vi "DeleteDVR.vi"(8 "error in (no error)":errorcluster, 10 "Error Return Notifier":refnum<notifier>, 11 "IAmGLF To Create DVR":refnum<class "IAmGLF.lvclass">) -> (0 "error out":errorcluster)   [LabVIEW 2024, in "GLF.lvlib" / "DVRHandler.lvlib"]
uses:
  DVRHandler.lvlib
  Action--enum.ctl
  IAmGLF/IAmGLF.lvclass
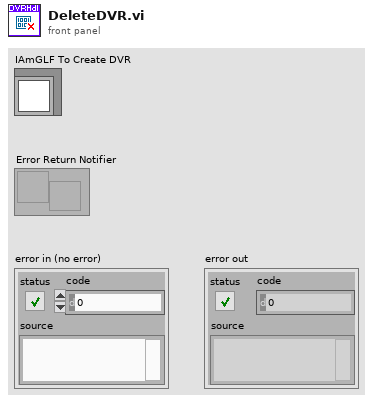
[diagram p1: front panel]
types:
  T1 = typedef "GLF.lvlib/DVRHandler.lvlib/Action--enum.ctl" = enum16{"Set IAmEngine", "Create DVR", "Delete DVR"}
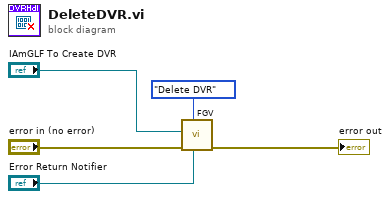
[diagram p0: block diagram]
diagram:
  n1 = call "FGV.vi"("Error Return Notifier"="Error Return Notifier", "Action"=Action--enum."Delete DVR", "error in (no error)"="error in (no error)", "IAmGLF To Create DVR"="IAmGLF To Create DVR") -> ("error out"=→"error out":errorcluster)  [unwired: 7 in]
